vi "cleanup.vi"(4 "error in (no error)":errorcluster, 5 "py interface file":path, 6 "Request data":variant, 7 "Python session in":refnum<k35>) -> (0 "error out":errorcluster, 2 "Response data":variant, 3 "Python session out":refnum<k35>)   [LabVIEW 2022 SP3]
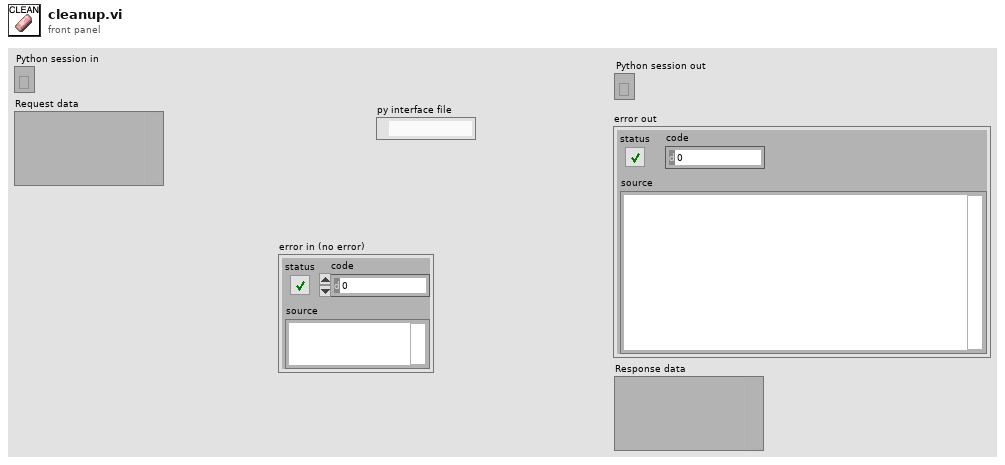
[diagram p1: front panel]
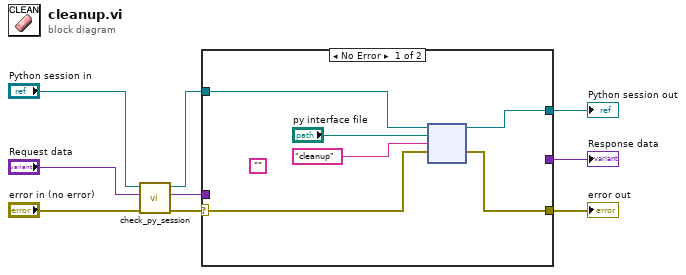
[diagram p0: block diagram]
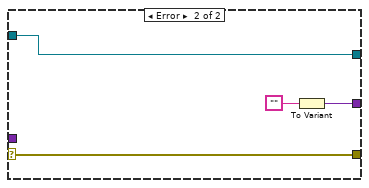
[diagram p2: hidden frame]
diagram:
  n1 = call "check_py_session.vi"("error in"="error in (no error)", "Request data"="Request data", "Python session in"="Python session in") -> ("error out"=w3:errorcluster, "Response data"=w4:variant, "Python session out"=w5:refnum<k35>)  [unwired: 2 in]
  n2 = case shown="No Error" w3 {
    selector: w3 -> [w10 w19]
    tunnel: w5 -> [w15 w18]
    tunnel: [w13 w18] -> w9
    tunnel: w4 -> [_ _]
    tunnel: [w12 w19] -> w2
    tunnel: [_ w16] -> w1
    frame No Error {
      (unwired) ""
      n3 = node(w15, "py interface file", "cleanup" ("function name"), w10) -> (w13:refnum<k35>, w12:errorcluster)  [unwired: 2 in, 2 out]
    }
    frame Error {
      n4 = To Variant(anything="") -> (Variant=w16:variant)
    }
  }
  "error out" <- w2
  "Python session out" <- w9
  "Response data" <- w1
